vi "OriginalDigitizerLive - Copy (2).vi"() -> ()   [LabVIEW 2020]
doc: "Example Description:\nThis example demonstrates how to enable Time Interleaved Sampling with the NI 5772 adapter module to achieve a sampling rate of 1.6GS/s. This example continuously acquires records of analog input data from the NI 5772 adapter module. It allows you to select an AI channel, trigger type, and record size. This VI must be compiled before it is run. \n\nRunning the VI:\nThis VI must be run from the NI 5772 - Getting Started (Host).vi. Refer to the host VI documentation for steps regarding running and configuring the FPGA VI. \n\nExecution Steps:\nRefer to the Block Diagram of this VI for execution comments."
uses:
  Controls/AI Trigger Type.ctl
  Controls/Aquire State.ctl
  Controls/NeighbouringAvgStates.ctl
  <vilib>/Platform/TimedLoop/XDataNode/timing_clust.ctl
  <vilib>/Platform/TimedLoop/XDataNode/nitl_modes.ctl
  <vilib>/Platform/TimedLoop/XDataNode/wakeup.ctl
  <vilib>/rvi/Emulation/niFpgaGetClockAttributes.vi
  <vilib>/rvi/Emulation/niFpgaSctlEmulationGetInTimedLoop.vi
  <vilib>/rvi/Emulation/niFpgaEmulationReportErrorSimple.vi
  <vilib>/rvi/Emulation/niFpgaProcessEmulError.vi
  <vilib>/rvi/eio/common/nirviEmuTemplateMethod_errors.vi
  <vilib>/rvi/Emulation/niFpgaCriticalErrorInLSC.vi
  <vilib>/rvi/interface/RandomDataEmulation/niFpgaRandomDataHandleErrors.vi
  <vilib>/rvi/Emulation/niFpgaEmulationIsFPGAContextNoSignature.vi
  <vilib>/rvi/errors/niFpgaSetErrorForExecOnDevCompSimple.vi
  <vilib>/rvi/eio/common/nirviEmuReportErrorAndStop.vi
  <vilib>/rvi/DataTransferAndStorage/Container/Common/niFpgaContainerGetUniqueNameForEmu.vi
  <vilib>/rvi/FIFO/Fifo_Resource/nirvififoEmulationSetSize.vi
  <vilib>/rvi/FIFO/Fifo_Resource/nirviFifoEmulationQueueMgr.vi
  <instcachedir>/0/nirviFifoEmulationQueueMgr_E5CAEC123FF24DC58D834DCA3CDAA9B5.lvgen/nirviFifoEmulationQueueMgr_E5CAEC123FF24DC58D834DCA3CDAA9B5_000.vi
  <vilib>/Utility/error.llb/Clear Errors.vi
  <vilib>/rvi/FIFO/Fifo_Resource/nirvififoEmulationCreateLock.vi
  <vilib>/rvi/FIFO/Fifo_Resource/nirvififoEmulationObtainLock.vi
  <vilib>/rvi/FIFO/Fifo_Resource/nirvififoEmulationReleaseLock.vi
  <vilib>/rvi/occurrence/nirviWaitOnOccurrenceBase.vi
  <vilib>/rvi/errors/nirviReportUnexpectedCaseInternalError.vi
  <vilib>/rvi/errors/nirviReportUnexpectedCaseInternalError (U32).vi
  <vilib>/rvi/FIFO/Fifo_Resource/nirvififoEmulationDetermineInputValidOut.vi
  <vilib>/eio/EIONode/EIONode.xnode
  <vilib>/Platform/TimedLoop/XDataNode/XDataNode.xnode
  <vilib>/rvi/DataTransferAndStorage/Container/XNode/niFpgaContainer.xnode
  <vilib>/rvi/interface/RandomDataEmulation/nirviRandomDataFpgaReadWriteTemplate.vi
  <vilib>/rvi/FIFO/Fifo_Resource/nirvififoEmulationRead.vi
  <vilib>/rvi/FIFO/Fifo_Resource/nirvififoEmulationWrite.vi
  <vilib>/Platform/TimedLoop/XDataNode/XDNodeRunTimeDep.lvlib
  <instrlib>/_niInstr/Basic Elements/v1/FPGA/niInstr Basic Elements v1 FPGA.lvlib
  Controls/DigitizerState.ctl
  <vilib>/rvi/Memory/Memory_Emulation/nirvimemoryEmulation.vi
  <vilib>/rvi/Memory/Memory_Emulation/nirvimemoryFastEmulation.vi
panel:
  in  "Recording":bool
  in  "WaitForWave\nCompletion [cycles]":u16
  out "F to H FIFO Overflow?":bool caption="FIFO Overflow?"
  out "AvgCount":u16=1
  in  "AvgCount_powerOf2":i16=1
  in  "DS":u8
  in  "Trigger":bool=TRUE
  out "Acquire State":T1
  in  "Delay Cycles":u16=512 caption="Samples Per Trigger" min=1 step=1
  out "TS FIFO In Overflow?":bool caption="FIFO Overflow?"
  in  "Samples Per Trigger":u16=512 min=1 step=1
  in  "Arm Trigger":bool
  in  "User Command Commit":bool
  in  "User Command":u8
  out "User Command Idle":bool
  out "User Command Status":u8
  in  "User Data 0":u16
  in  "User Data 1":u8
  out "PLL Locked":bool
  out "User Error":bool
  out "Configured?":bool
  out "DMA FIFO Overflow?":bool caption="FIFO Overflow?"
  in  "Trigger Level":i16
  in  "Trigger Type":T2
  # "Resource Configuration"
  # "Refer to the Block Diagram of this VI for execution comments."
  # "For other instructions, select Help>>Show Context Help and move the cursor over the VI icon to display help for this VI."
  # "Analog Input"
  # "Clock Configuration"
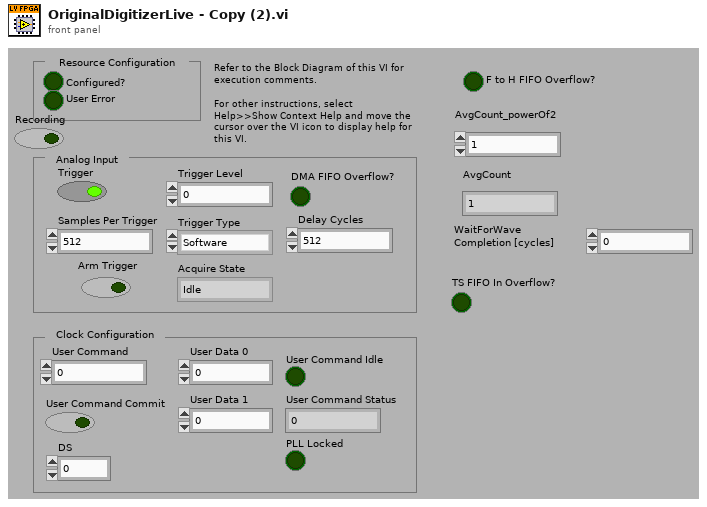
[diagram p1: front panel]
types:
  T1 = typedef "Aquire State.ctl" = enum8{"Idle", "Wait for Trigger", "AlignWave", "Hold Aquire", "Acquire", "WaitForWaveCompletion", "CheckAvg"}
  T2 = typedef "AI Trigger Type.ctl" = enum8{"Software", "Data Edge"}
  T3 = typedef "NeighbouringAvgStates.ctl" = enum16{"Read_noDS", "Write1_noDS", "Write2_noDS"}
  T4 = typedef "DigitizerState.ctl" = enum16{"Init", "Build/Clear Accumulator", "GetData", "SetData", "AverageCountCheck", "SendtoHost"}
  T5 = typedef "XDNodeRunTimeDep.lvlib/timing_clust.ctl" = cluster{"Expected End [f-1]":u64, "Actual End [f-1]":u64, "Finished Late? [f-1]":bool, "Expected End [i-1]":u64, "Actual End [i-1]":u64, "Finished Late? [i-1]":bool, "Expected Start [i]":u64, "Actual Start [i]":u64, "Expected Start [f]":u64, "Actual Start [f]":u64, "Source Name":string, "Structure Name":string, "Period":i64, "Deadline":i64, "Offset":i64, "Start":i64, "Priority":i32, "Timeout":i32, "Mode":T6, "Wakeup Reason":T7, "Error":errorcluster, "Source Type":string, "Secondary Source Type":string, "Global End Time":u64, "Global Start Time":u64, "Frame Duration":u64, "Iteration Duration":u64, "Assigned CPU":i32, "I/O Scan Engine Mode":u32}
  T6 = typedef "XDNodeRunTimeDep.lvlib/nitl_modes.ctl" = enum32{"No Change", "Process missed periods, maintain original phase", "Discard missed periods, maintain original phase", "Process missed periods, ignore original phase", "Discard missed periods, ignore original phase"}
  T7 = typedef "XDNodeRunTimeDep.lvlib/wakeup.ctl" = enum32{"Normal", "Aborted", "Asynchronous wakeup", "Timing source error", "Timed loop error", "Timeout"}
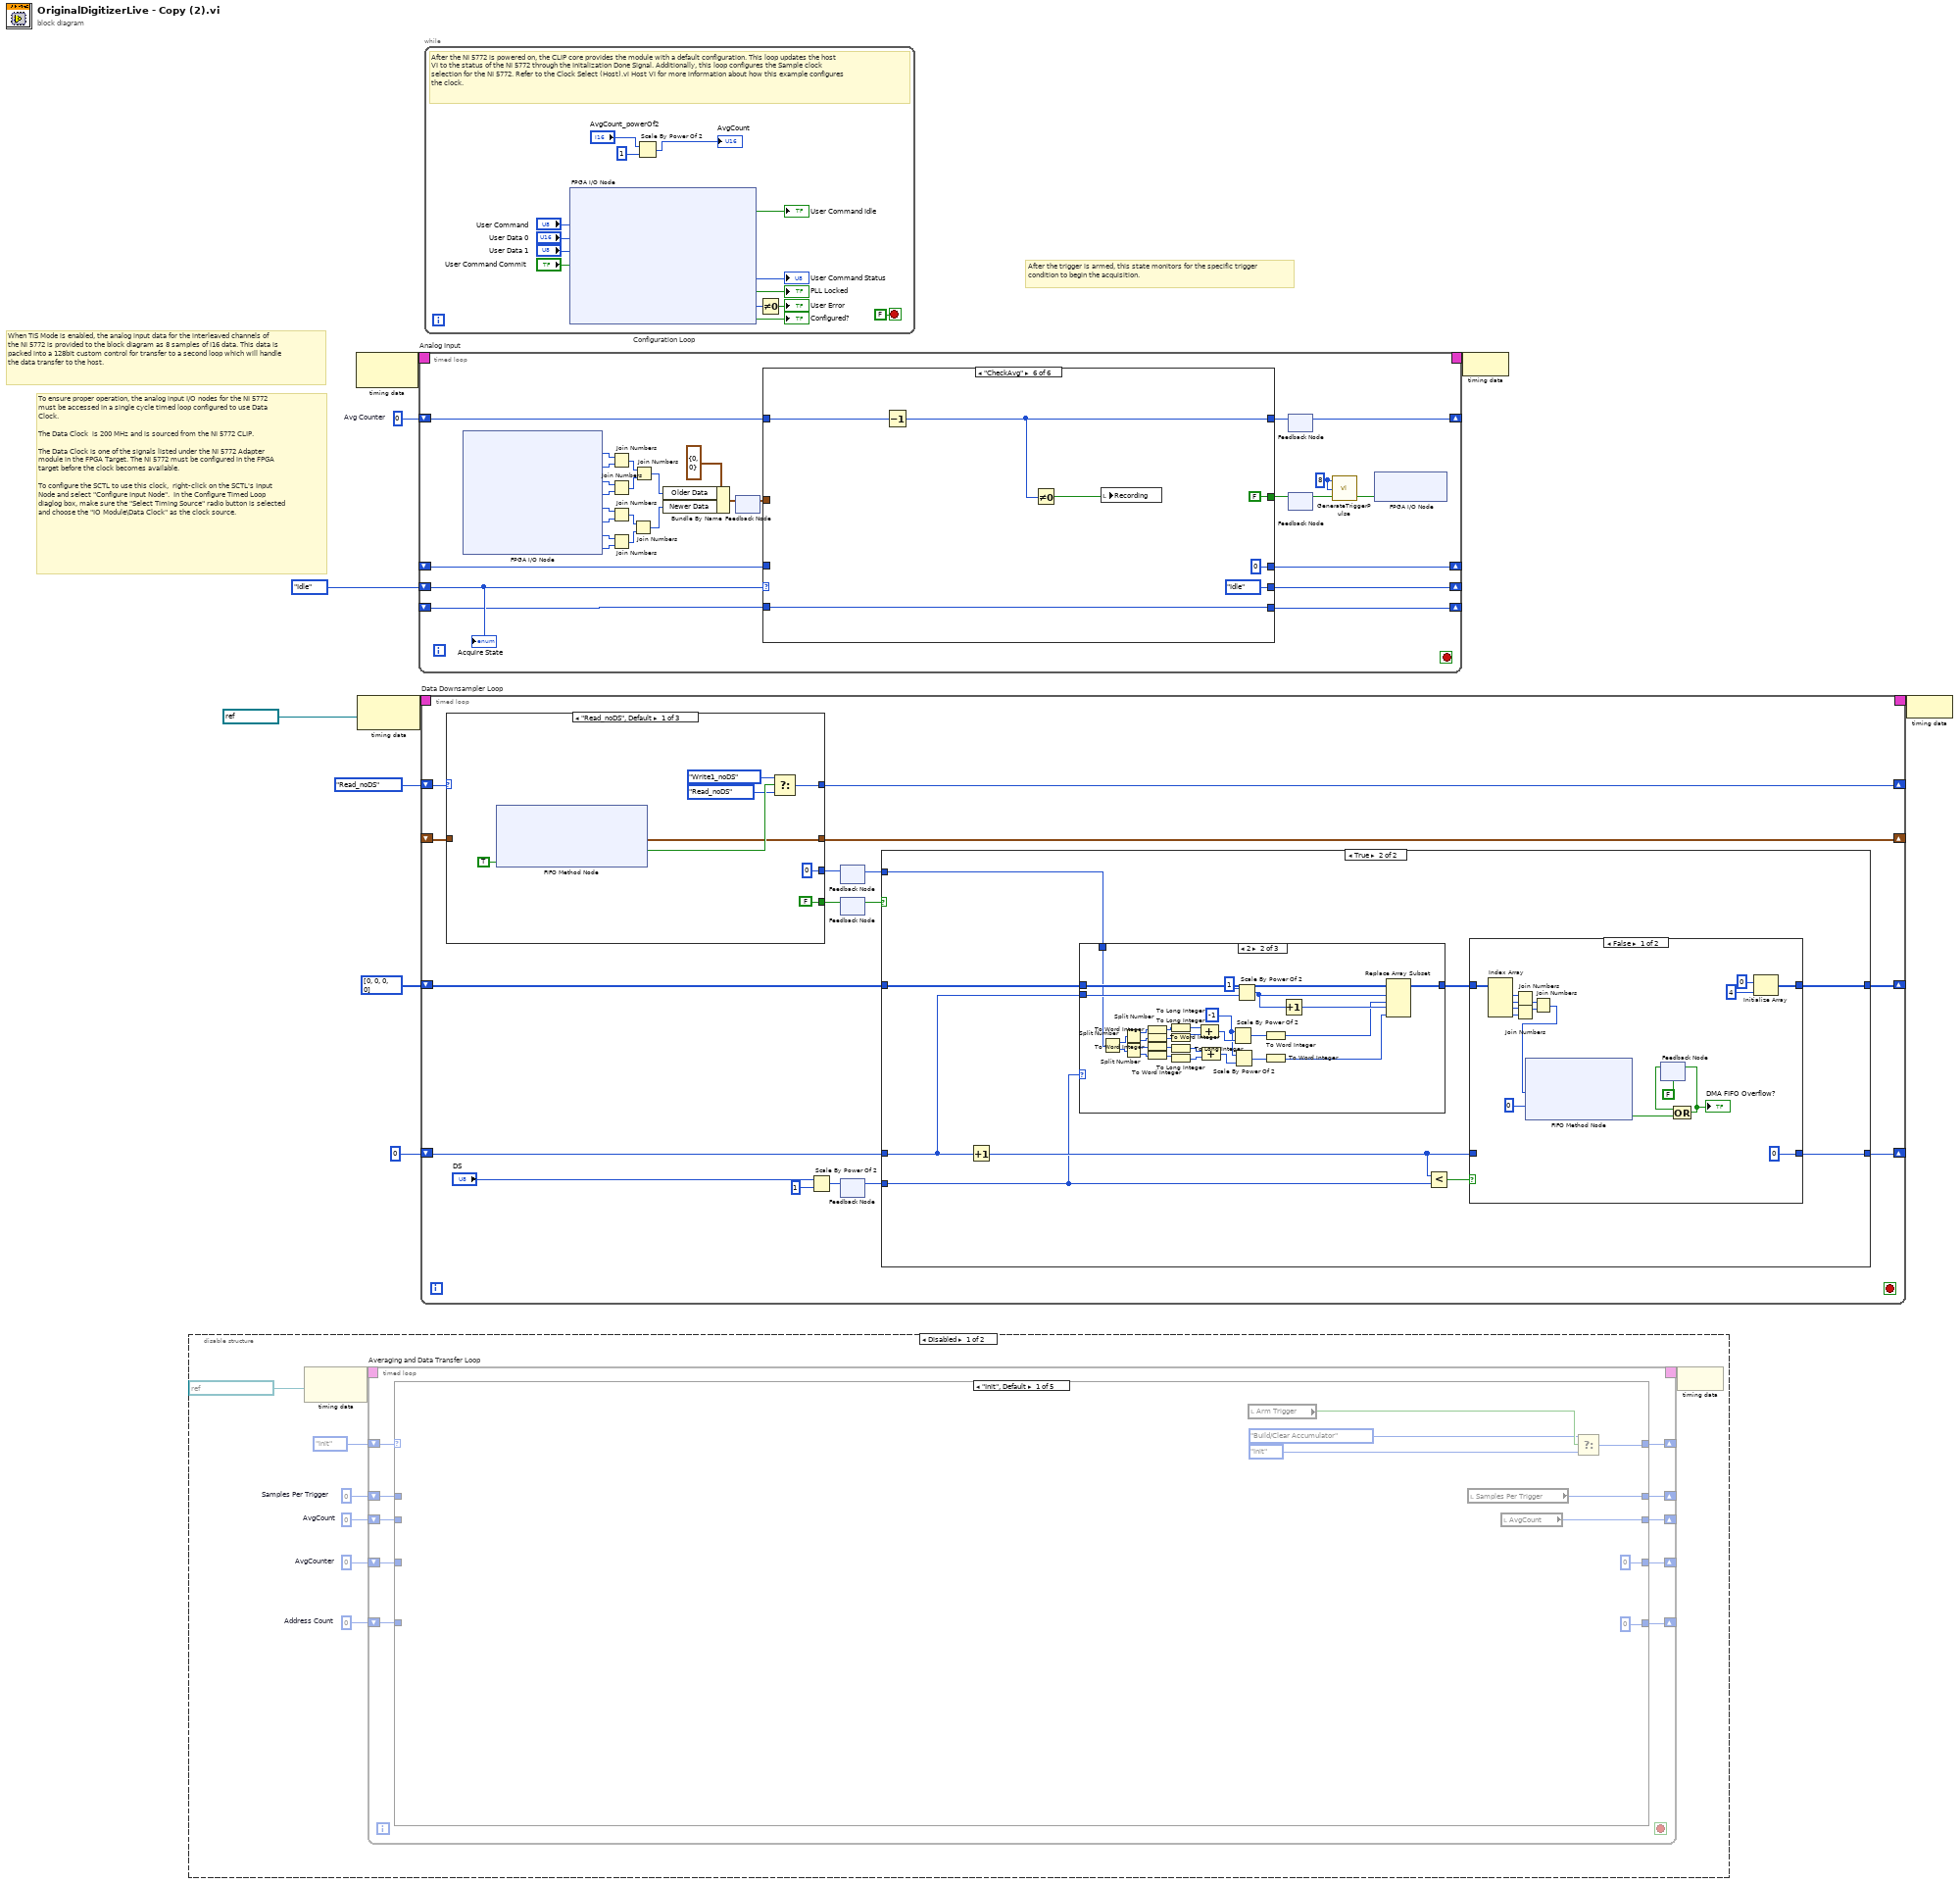
[diagram p0: block diagram]
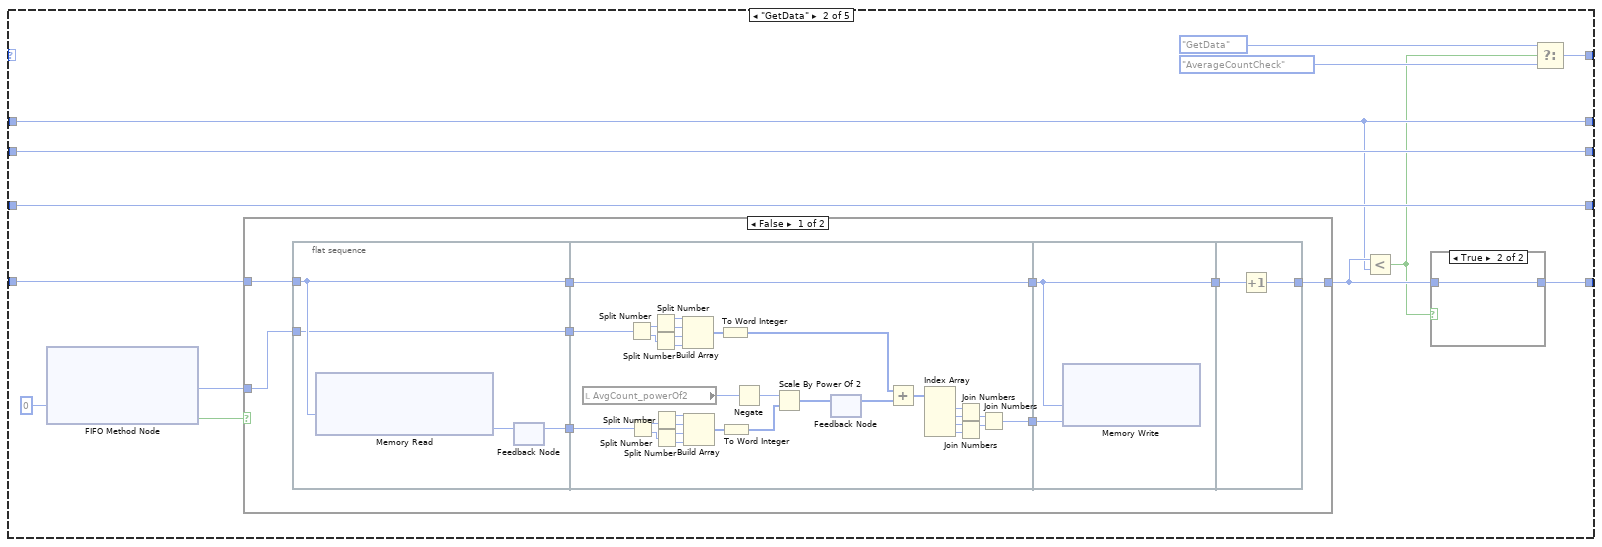
[diagram p2: hidden frame]
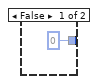
[diagram p3: hidden frame]
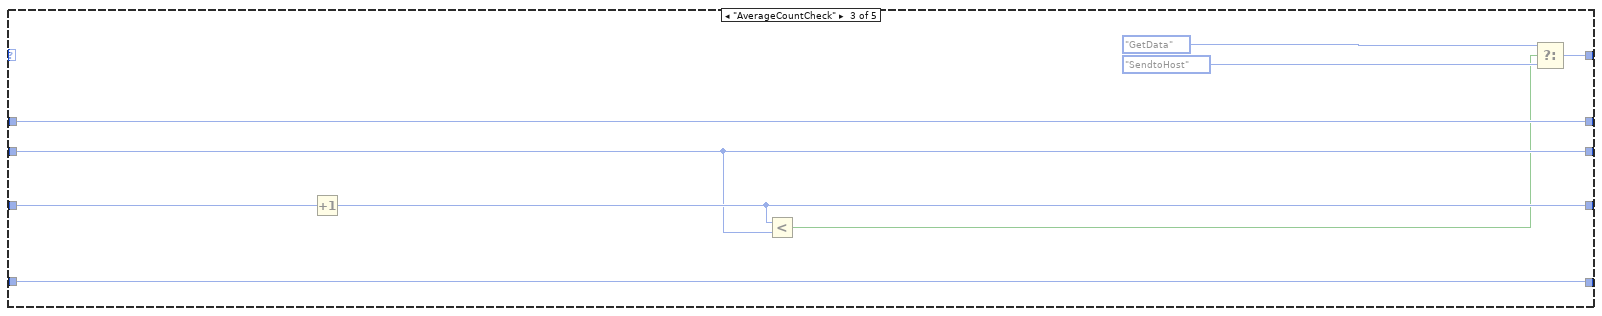
[diagram p5: hidden frame]
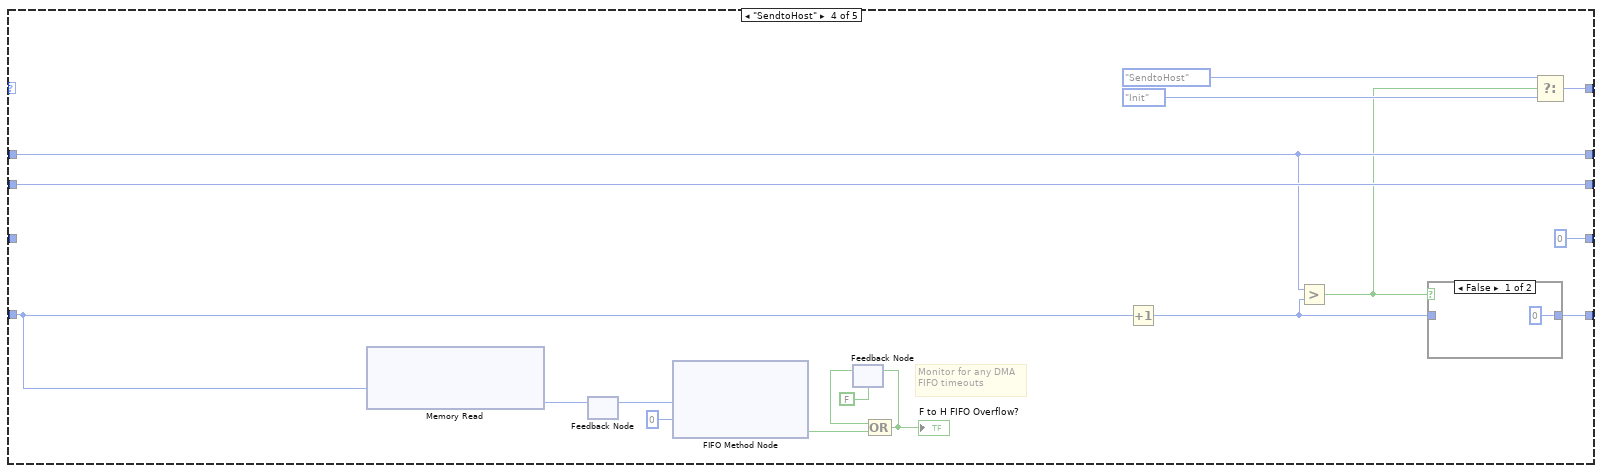
[diagram p6: hidden frame]
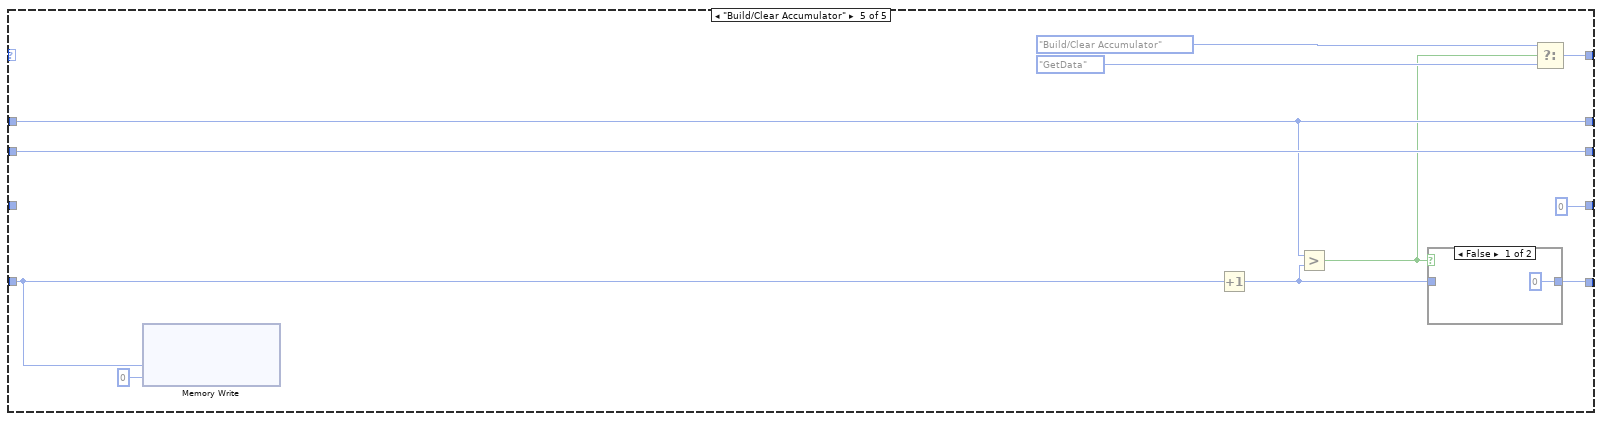
[diagram p8: hidden frame]
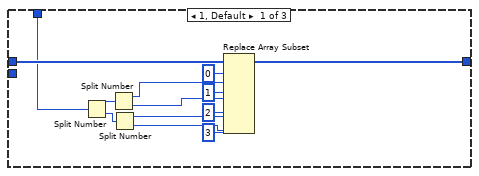
[diagram p13: hidden frame]
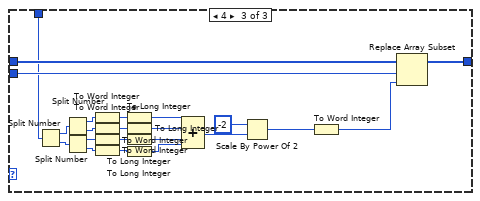
[diagram p14: hidden frame]
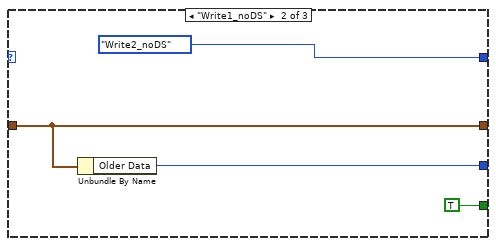
[diagram p15: hidden frame]
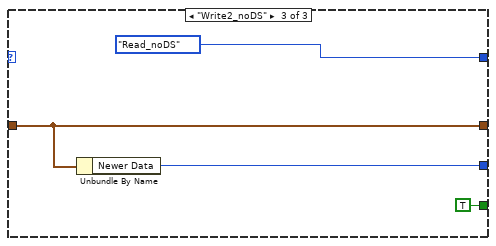
[diagram p16: hidden frame]
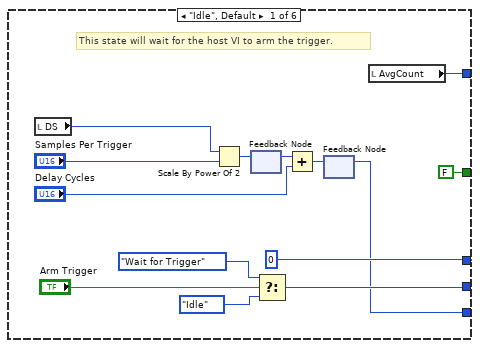
[diagram p17: hidden frame]
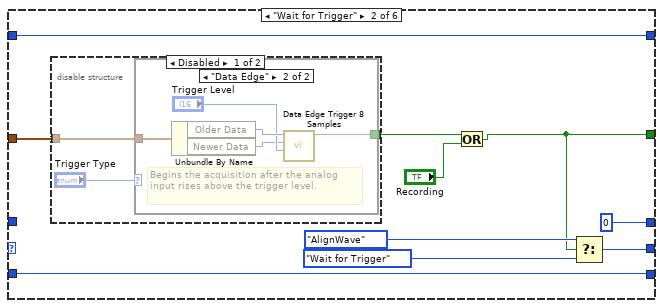
[diagram p18: hidden frame]
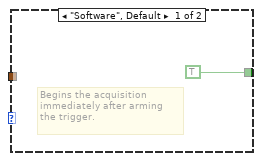
[diagram p19: hidden frame]
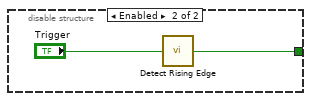
[diagram p20: hidden frame]
diagram:
  w1 = u16 0  # Avg Counter
  # "After the trigger is armed, this state monitors for the specific trigger condition to begin the acquisition."
  # "When TIS Mode is enabled, the analog input data for the interleaved channels of the NI 5772 is provided to the block diagram as 8 samples of I16 data. This data is packed into a 128bit custom control for transfer to a second loop which will handle the data transfer to the host."
  # "To ensure proper operation, the analog input I/O nodes for the NI 5772 must be accessed in a single cycle timed loop configured to use Data Clock. \n\nThe Data Clock  is 200 MHz and is sourced from the NI 5772 CLIP.\n\nThe Data Clock is one of the signals listed under the NI 5772 Adapter module in the FPGA Target. The NI 5772 must be configured in the FPGA target before the clock becomes available. \n\nTo configure the SCTL to use this clock,  right-click on the SCTL's Input Node and select \"Configure Input Node\".  In the Configure Timed Loop diaglog box, make sure the \"Select Timing Source\" radio button is selected and choose the \"IO Module\\Data Clock\" as the clock source."
  n1 = disable-structure shown="Disabled" {
    frame Disabled {
      w16 = u16 0  # AvgCounter
      w15 = u32 0  # Address Count
      w14 = u16 0  # AvgCount
      w13 = u16 0  # Samples Per Trigger
      n2 = node-c288(refnum<k21> "200 MHz Clock" ("Source Name")) -> (w18:T5)
      n3 = timed-loop "Averaging and Data Transfer Loop" {
        timing: w18 -> [_]
        timing-out: [_] -> w17
        shift-right: [w27] -> _
        shift-left: DigitizerState."Init" -> [w28]
        shift-right: [w26] -> _
        shift-left: w13 -> [w24]
        shift-right: [w25] -> _
        shift-left: w14 -> [w23]
        shift-right: [w21] -> _
        shift-left: w15 -> [w22]
        shift-right: [w19] -> _
        shift-left: w16 -> [w20]
        stop <- _ stop-if-true
        n4 = case shown="\"Init\", Default" w28 {
          tunnel: [w32 w47 w107 w123 w136] -> w27
          tunnel: [w30 w39 w105 w121 w134] -> w26
          tunnel: [w33 w46 w102 w126 w139] -> w25
          tunnel: w24 -> [_ w39 w105 w121 w134]
          tunnel: w23 -> [_ w46 w102 w126 w139]
          tunnel: w22 -> [_ w42 w106 w111 w130]
          tunnel: [u32 0 w41 w106 w122 w135] -> w21
          tunnel: [u16 0 w44 w103 u16 0 ("AvgCounter") u16 0 ("AvgCounter")] -> w19
          tunnel: w20 -> [_ w44 w104 _ _]
          frame "Init", Default {
            n5 = local read "Arm Trigger"() -> (w36:bool)
            n6 = local read "Samples Per Trigger"() -> (w30:u16)
            n7 = local read "AvgCount"() -> (w33:u16)
            n8 = Select(t=DigitizerState."Build/Clear Accumulator", s=w36, f=DigitizerState."Init") -> (s? t:f=w32:T4)
          }
          frame "GetData" {
            n9 = xnode ("FIFO Method Node")("Timeout"=0) -> ("Element"=w43:u64, "Timed Out?"=w38:bool)  [unwired: 1 in, 1 out]
            n10 = case shown="False" w38 {
              tunnel: w43 -> [w57 _]
              tunnel: w42 -> [w59 w100]
              tunnel: [w56 w100] -> w40
              frame False {
                n11 = flat-sequence {
                  tunnel: [w63] -> w60
                  tunnel: w59 -> [w62]
                  tunnel: w57 -> [w61]
                  tunnel: [w62] -> w55
                  tunnel: [w61] -> w53
                  tunnel: w60 -> [w66]
                  tunnel: [w85] -> w58
                  tunnel: w55 -> [w84]
                  tunnel: [w84] -> w54
                  tunnel: w53 -> [w75]
                  tunnel: w58 -> [w97]
                  tunnel: w54 -> [w96]
                  tunnel: [w96] -> w52
                  tunnel: [w98] -> w56
                  tunnel: w52 -> [w99]
                  frame #0 {
                    n12 = xnode ("Memory Read")("Address"=w62) -> ("Data"=w64:u64)  [unwired: 1 in, 1 out]
                    n13 = feedback #1() -> (w63:u64)  [unwired: 1 in]
                    n14 = feedback-in #1(w64) -> ()
                  }
                  frame #1 {
                    n15 = local read "AvgCount_powerOf2"() -> (w94:i16)
                    n16 = Split Number(x=w75) -> (hi(x)=w82:u32, lo(x)=w81:u32)
                    n17 = Split Number(x=w66) -> (hi(x)=w67:u32, lo(x)=w68:u32)
                    n18 = Split Number(x=w82) -> (hi(x)=w80:u16, lo(x)=w79:u16)
                    n19 = Split Number(x=w81) -> (hi(x)=w78:u16, lo(x)=w77:u16)
                    n20 = Split Number(x=w67) -> (hi(x)=w69:u16, lo(x)=w70:u16)
                    n21 = Split Number(x=w68) -> (hi(x)=w71:u16, lo(x)=w72:u16)
                    n22 = Build Array(w80, w79, w78, w77) -> (w76:u16[])
                    n23 = Build Array(w69, w70, w71, w72) -> (w73:u16[])
                    n24 = To Word Integer(number=w76) -> (16bit integer=w74:i16[])
                    n25 = To Word Integer(number=w73) -> (16bit integer=w65:i16[])
                    n26 = Negate(x=w94) -> (-x=w95:i16)
                    n27 = Scale By Power Of 2(n=w95, x=w65) -> (x*2^n=w93:i16[])
                    n28 = feedback-in #2(w93) -> ()
                    n29 = feedback #2() -> (w83:i16[])  [unwired: 1 in]
                    n30 = Add(x=w74, y=w83) -> (x+y=w86:i16[])
                    n31 = Index Array(array=w86) -> (element #1=w89:i16, element #2=w90:i16, element #3=w91:i16, element #4=w92:i16)  [unwired: 4 in]
                    n32 = Join Numbers(hi=w89, lo=w90) -> ((hi.lo)=w87:u32)
                    n33 = Join Numbers(hi=w91, lo=w92) -> ((hi.lo)=w88:u32)
                    n34 = Join Numbers(hi=w87, lo=w88) -> ((hi.lo)=w85:u64)
                  }
                  frame #2 {
                    n35 = xnode ("Memory Write")("Address"=w96, "Data"=w97) -> ()  [unwired: 1 in, 1 out]
                  }
                  frame #3 {
                    n36 = Increment(x=w99) -> (x+1=w98:u32)
                  }
                }
              }
              frame True {
              }
            }
            n37 = Less?(x=w40, y=w39) -> (x < y?=w37:bool)
            n38 = case shown="True" w37 {
              tunnel: w40 -> [_ w51]
              tunnel: [u32 0 w51] -> w41
              frame False {
              }
              frame True {
              }
            }
            n39 = Select(t=DigitizerState."GetData", s=w37, f=DigitizerState."AverageCountCheck") -> (s? t:f=w47:T4)
          }
          frame "AverageCountCheck" {
            n40 = Increment(x=w104) -> (x+1=w103:u16)
            n41 = Less?(x=w103, y=w102) -> (x < y?=w101:bool)
            n42 = Select(t=DigitizerState."GetData", s=w101, f=DigitizerState."SendtoHost") -> (s? t:f=w107:T4)
          }
          frame "SendtoHost" {
            # "Monitor for any DMA FIFO timeouts"
            n43 = xnode ("Memory Read")("Address"=w111) -> ("Data"=w112:u64)  [unwired: 1 in, 1 out]
            n44 = feedback #3() -> (w110:u64)  [unwired: 1 in]
            n45 = feedback-in #3(w112) -> ()
            n46 = xnode ("FIFO Method Node")("Element"=w110, "Timeout"=0) -> ("Timed Out?"=w117:bool)  [unwired: 1 in, 1 out]
            n47 = feedback #4(FALSE) -> (w116:bool)
            n48 = Compound Arithmetic op=OR(w116, w117) -> (w118:bool)
            "F to H FIFO Overflow?" <- w118
            n49 = feedback-in #4(w118) -> ()
            n50 = Increment(x=w111) -> (x+1=w120:u32)
            n51 = Greater?(x=w121, y=w120) -> (0:w119:bool)
            n52 = case shown="False" w119 {
              tunnel: w120 -> [_ w128]
              tunnel: [u32 0 w128] -> w122
              frame False {
              }
              frame True {
              }
            }
            n53 = Select(t=DigitizerState."SendtoHost", s=w119, f=DigitizerState."Init") -> (s? t:f=w123:T4)
          }
          frame "Build/Clear Accumulator" {
            n54 = xnode ("Memory Write")("Address"=w130, "Data"=u64 0) -> ()  [unwired: 1 in, 1 out]
            n55 = Increment(x=w130) -> (x+1=w133:u32)
            n56 = Greater?(x=w134, y=w133) -> (0:w132:bool)
            n57 = case shown="False" w132 {
              tunnel: w133 -> [_ w141]
              tunnel: [u32 0 w141] -> w135
              frame False {
              }
              frame True {
              }
            }
            n58 = Select(t=DigitizerState."Build/Clear Accumulator", s=w132, f=DigitizerState."GetData") -> (s? t:f=w136:T4)
          }
        }
      }
      n59 = node-c288(w17) -> ()
    }
    frame Enabled {
    }
  }
  n60 = node-c288() -> (w10:T5)  [unwired: 1 in]
  n61 = node-c288(refnum<k21> "160MHz" ("Source Name")) -> (w6:T5)
  n62 = timed-loop "Analog Input" {
    timing: w10 -> [_]
    timing-out: [_] -> w9
    shift-right: [w176] -> _
    shift-left: Aquire_State."Idle" ("Acquire State") -> [w166]
    shift-right: [w177] -> _
    shift-left: _ -> [w167]
    shift-right: [w175] -> _
    shift-left: _ -> [w165]
    shift-right: [w148] -> _
    shift-left: w1 -> [w151]
    stop <- _ stop-if-true
    w153 = u16 8 ("Pulse Width On [cycles]")
    n63 = xnode "FPGA I/O Node"() -> ("IO Module\\AI 1 Data N-3"=w158:i16, "IO Module\\AI 0 Data N-3"=w157:i16, "IO Module\\AI 1 Data N-2"=w156:i16, "IO Module\\AI 0 Data N-2"=w155:i16, "IO Module\\AI 1 Data N-1"=w159:i16, "IO Module\\AI 0 Data N-1"=w160:i16, "IO Module\\AI 1 Data N"=w161:i16, "IO Module\\AI 0 Data N"=w162:i16)  [unwired: 8 in, 8 out]
    n64 = Join Numbers(hi=w158, lo=w157) -> ((hi.lo)=w170:u32)
    n65 = Join Numbers(hi=w156, lo=w155) -> ((hi.lo)=w172:u32)
    n66 = Join Numbers(hi=w159, lo=w160) -> ((hi.lo)=w171:u32)
    n67 = Join Numbers(hi=w161, lo=w162) -> ((hi.lo)=w173:u32)
    n68 = Join Numbers(hi=w171, lo=w173) -> ((hi.lo)=w163:u64)
    n69 = Join Numbers(hi=w170, lo=w172) -> ((hi.lo)=w164:u64)
    n70 = Bundle By Name(cluster=cluster{"Older Data":u64, "Newer Data":u64} {"Older Data"=0, "Newer Data"=0} ("Element"), "Older Data"=w164, "Newer Data"=w163) -> (w168:cluster{"Older Data":u64, "Newer Data":u64})
    n71 = feedback #5() -> (w174:cluster{"Older Data":u64, "Newer Data":u64})  [unwired: 1 in]
    n72 = feedback-in #5(w168) -> ()
    n73 = case shown="\"CheckAvg\"" w166 {
      tunnel: [u16 0 u16 0 w217 w226 w249 u16 0 ("f")] -> w177
      tunnel: w167 -> [_ _ w217 w240 w247 _]
      tunnel: [w188 w197 w218 w239 w244 Aquire_State."Idle" ("Acquire State")] -> w176
      tunnel: [w185 w201 w216 w236 w250 w256] -> w175
      tunnel: w165 -> [_ w201 w216 w236 w250 w256]
      tunnel: w174 -> [_ w200 _ w235 _ _]
      tunnel: [FALSE ("edge detected") w193 FALSE ("edge detected") FALSE ("edge detected") FALSE ("edge detected") FALSE ("edge detected")] -> w152
      tunnel: w151 -> [_ w194 w214 w222 w242 w257]
      tunnel: [w179 w194 w214 w222 w242 w254] -> w150
      frame "Idle", Default {
        # "This state will wait for the host VI to arm the trigger."
        n74 = local read "DS"() -> (w181:u8)
        n75 = Scale By Power Of 2(n=w181, x="Samples Per Trigger") -> (x*2^n=w183:u16)
        n76 = feedback-in #6(w183) -> ()
        n77 = feedback #6() -> (w180:u16)  [unwired: 1 in]
        n78 = Select(t=Aquire_State."Wait for Trigger" ("Acquire State"), s="Arm Trigger", f=Aquire_State."Idle" ("Acquire State")) -> (s? t:f=w188:T1)
        n79 = Add(x=w180, y="Delay Cycles") -> (x+y=w186:u16)
        n80 = feedback-in #7(w186) -> ()
        n81 = feedback #7() -> (w185:u16)  [unwired: 1 in]
        n82 = local read "AvgCount"() -> (w179:u16)
      }
      frame "Wait for Trigger" {
        n83 = disable-structure shown="Disabled" {
          disable-tunnel: w200 -> [w203 _]
          disable-tunnel: [w202 w211] -> w195
          frame Disabled {
            n84 = case shown="\"Data Edge\"" "Trigger Type" {
              tunnel: w203 -> [_ w210]
              tunnel: [TRUE ("Trigger") w209] -> w202
              frame "Software", Default {
                # "Begins the acquisition immediately after arming the trigger."
              }
              frame "Data Edge" {
                # "Begins the acquisition after the analog input rises above the trigger level."
                n85 = Unbundle By Name(w210) -> ("Older Data"=w208:u64, "Newer Data"=w206:u64)
                n86 = call "Data Edge Trigger 8 Samples.vi"("Trigger Level"="Trigger Level", "Newer Data In"=w206, "Older Data In"=w208) -> ("Trigger"=w209:bool)  [unwired: 8 in]
              }
            }
          }
          frame Enabled {
            n87 = call <instrlib>:"Detect Rising Edge.vi"("signal"="Trigger") -> ("edge detected"=w211:bool)  [unwired: 14 in]
          }
        }
        n88 = Or(x=w195, y="Recording") -> (x .or. y?=w193:bool)
        n89 = Select(t=Aquire_State."AlignWave" ("Acquire State"), s=w193, f=Aquire_State."Wait for Trigger") -> (s? t:f=w197:T1)
      }
      frame "AlignWave" {
        n90 = xnode "FPGA I/O Node"() -> ("PXI_Trig0"=w215:bool)  [unwired: 1 in, 1 out]
        n91 = Select(t=Aquire_State."Acquire" ("Acquire State"), s=w215, f=Aquire_State."AlignWave") -> (s? t:f=w218:T1)
      }
      frame "Acquire" {
        # "Monitor for any  FIFO timeouts"
        # "While in this state, data is pushed into a DMA FIFO until the desired number of samples per record have been acquired."
        n92 = local read "Delay Cycles"() -> (w234:u16)
        n93 = Increment(x=w240) -> (x+1=w225:u16)
        n94 = Less?(x=w234, y=w225) -> (x < y?=w230:bool)
        n95 = feedback-in #8(w230) -> ()
        n96 = feedback #8() -> (w227:bool)  [unwired: 1 in]
        n97 = Less?(x=w225, y=w236) -> (x < y?=w224:bool)
        n98 = xnode ("FIFO Method Node")("Element"=w235, "Input Valid"=w227) -> ("Ready for Input"=w229:bool)  [unwired: 1 in, 1 out]
        n99 = Not(x=w229) -> (.not. x?=w228:bool)
        n100 = feedback #9(FALSE) -> (w231:bool)
        n101 = Or(x=w231, y=w228) -> (x .or. y?=w232:bool)
        "TS FIFO In Overflow?" <- w232
        n102 = feedback-in #9(w232) -> ()
        n103 = Select(t=Aquire_State."Acquire" ("Acquire State"), s=w224, f=Aquire_State."WaitForWaveCompletion" ("Acquire State")) -> (s? t:f=w239:T1)
        n104 = Select(t=w225, s=w224, f=u16 0) -> (s? t:f=w226:u16)
      }
      frame "WaitForWaveCompletion" {
        n105 = Greater?(x="WaitForWave\nCompletion [cycles]", y=w247) -> (0:w243:bool)
        n106 = Increment(x=w247) -> (x+1=w249:u16)
        n107 = Select(t=Aquire_State."WaitForWaveCompletion" ("Acquire State"), s=w243, f=Aquire_State."CheckAvg" ("Acquire State")) -> (s? t:f=w244:T1)
      }
      frame "CheckAvg" {
        n108 = Decrement(x=w257) -> (x-1=w254:u16)
        n109 = Not Equal To 0?(x=w254) -> (x != 0?=w252:bool)
        n110 = local write "Recording"(w252) -> ()
      }
    }
    n111 = feedback-in #10(w150) -> ()
    n112 = feedback #10() -> (w148:u16)  [unwired: 1 in]
    n113 = feedback-in #11(w152) -> ()
    n114 = feedback #11() -> (w149:bool)  [unwired: 1 in]
    n115 = call "GenerateTriggerPulse.vi"("Trigger"=w149, "Pulse Width Off [cycles]"=w153, "Pulse Width On [cycles]"=w153) -> ("Out"=w154:bool)  [unwired: 2 out]
    n116 = xnode "FPGA I/O Node"("PXI_Trig1"=w154) -> ()  [unwired: 1 in, 1 out]
    "Acquire State" <- w166
  }
  n117 = timed-loop "Data Downsampler Loop" {
    shift-right: [w274] -> _
    shift-left: NeighbouringAvgStates."Read_noDS" -> [w275]
    timing: w6 -> [_]
    timing-out: [_] -> w5
    shift-right: [w273] -> _
    shift-left: _ -> [w272]
    shift-right: [w262] -> _
    shift-left: u16 0 -> [w263]
    shift-right: [w260] -> _
    shift-left: i16[] [0, 0, 0, 0] -> [w261]
    stop <- _ stop-if-true
    n118 = case shown="\"Read_noDS\", Default" w275 {
      tunnel: [w375 NeighbouringAvgStates."Write2_noDS" ("f") NeighbouringAvgStates."Read_noDS" ("f")] -> w274
      tunnel: [w371 w379 w383] -> w273
      tunnel: w272 -> [_ w379 w383]
      tunnel: [u64 0 ("Newer Data") w378 w382] -> w270
      tunnel: [FALSE ("Input Valid") TRUE ("Input Valid") TRUE ("Input Valid")] -> w271
      frame "Read_noDS", Default {
        n119 = xnode ("FIFO Method Node")("Ready for Output"=TRUE) -> ("Element"=w371:cluster{"Older Data":u64, "Newer Data":u64}, "Output Valid"=w374:bool)  [unwired: 1 in, 1 out]
        n120 = Select(t=NeighbouringAvgStates."Write1_noDS", s=w374, f=NeighbouringAvgStates."Read_noDS") -> (s? t:f=w375:T3)
      }
      frame "Write1_noDS" {
        n121 = Unbundle By Name(w379) -> ("Older Data"=w378:u64)
      }
      frame "Write2_noDS" {
        n122 = Unbundle By Name(w383) -> ("Newer Data"=w382:u64)
      }
    }
    n123 = Scale By Power Of 2(n="DS", x=u8 1) -> (x*2^n=w268:u8)
    n124 = feedback-in #12(w270) -> ()
    n125 = feedback #12() -> (w265:u64)  [unwired: 1 in]
    n126 = feedback-in #13(w271) -> ()
    n127 = feedback #13() -> (w264:bool)  [unwired: 1 in]
    n128 = feedback-in #14(w268) -> ()
    n129 = feedback #14() -> (w266:u8)  [unwired: 1 in]
    n130 = case shown="True" w264 {
      tunnel: w265 -> [_ w283]
      tunnel: w266 -> [_ w282]
      tunnel: w263 -> [w277 w281]
      tunnel: [w277 w280] -> w262
      tunnel: w261 -> [w276 w279]
      tunnel: [w276 w278] -> w260
      frame False {
      }
      frame True {
        n131 = Increment(x=w281) -> (x+1=w286:u16)
        n132 = case shown="2" w282 {
          tunnel: w279 -> [w318 w340 w362]
          tunnel: [w317 w339 w361] -> w285
          tunnel: w281 -> [_ w336 w360]
          tunnel: w283 -> [w306 w334 w355]
          frame 1, Default {
            n133 = Split Number(x=w306) -> (hi(x)=w316:u32, lo(x)=w315:u32)
            n134 = Split Number(x=w316) -> (hi(x)=w314:u16, lo(x)=w313:u16)
            n135 = Split Number(x=w315) -> (hi(x)=w312:u16, lo(x)=w311:u16)
            n136 = Replace Array Subset(array=w318, new element #1=w314, index #1=0 ("index"), new element #2=w313, index #2=1 ("index"), new element #3=w312, index #3=2 ("index"), new element #4=w311, index #4=3 ("index")) -> (w317:i16[])
          }
          frame 2 {
            w319 = i16 -1 ("n")
            n137 = Split Number(x=w334) -> (hi(x)=w346:u32, lo(x)=w345:u32)
            n138 = Split Number(x=w346) -> (hi(x)=w344:u16, lo(x)=w343:u16)
            n139 = Split Number(x=w345) -> (hi(x)=w342:u16, lo(x)=w341:u16)
            n140 = To Word Integer(number=w344) -> (16bit integer=w333:i16)
            n141 = To Word Integer(number=w343) -> (16bit integer=w331:i16)
            n142 = To Word Integer(number=w342) -> (16bit integer=w330:i16)
            n143 = To Word Integer(number=w341) -> (16bit integer=w332:i16)
            n144 = To Long Integer(number=w333) -> (32bit integer=w329:i32)
            n145 = To Long Integer(number=w331) -> (32bit integer=w328:i32)
            n146 = To Long Integer(number=w330) -> (32bit integer=w327:i32)
            n147 = To Long Integer(number=w332) -> (32bit integer=w326:i32)
            n148 = Compound Arithmetic op=ADD(w329, w328) -> (w320:i32)
            n149 = Compound Arithmetic op=ADD(w327, w326) -> (w321:i32)
            n150 = Scale By Power Of 2(n=w319, x=w320) -> (x*2^n=w322:i32)
            n151 = Scale By Power Of 2(n=w319, x=w321) -> (x*2^n=w323:i32)
            n152 = Scale By Power Of 2(n=i16 1, x=w336) -> (x*2^n=w337:u16)
            n153 = To Word Integer(number=w322) -> (16bit integer=w324:i16)
            n154 = To Word Integer(number=w323) -> (16bit integer=w325:i16)
            n155 = Increment(x=w337) -> (x+1=w338:u16)
            n156 = Replace Array Subset(array=w340, new element #1=w324, index #1=w337, new element #2=w325, index #2=w338) -> (w339:i16[])
          }
          frame 4 {
            n157 = Split Number(x=w355) -> (hi(x)=w368:u32, lo(x)=w367:u32)
            n158 = Split Number(x=w368) -> (hi(x)=w366:u16, lo(x)=w365:u16)
            n159 = Split Number(x=w367) -> (hi(x)=w364:u16, lo(x)=w363:u16)
            n160 = To Word Integer(number=w366) -> (16bit integer=w359:i16)
            n161 = To Word Integer(number=w365) -> (16bit integer=w358:i16)
            n162 = To Word Integer(number=w364) -> (16bit integer=w357:i16)
            n163 = To Word Integer(number=w363) -> (16bit integer=w356:i16)
            n164 = To Long Integer(number=w359) -> (32bit integer=w351:i32)
            n165 = To Long Integer(number=w358) -> (32bit integer=w352:i32)
            n166 = To Long Integer(number=w357) -> (32bit integer=w353:i32)
            n167 = To Long Integer(number=w356) -> (32bit integer=w354:i32)
            n168 = Compound Arithmetic op=ADD(w351, w352, w353, w354) -> (w350:i32)
            n169 = Scale By Power Of 2(n=i16 -2, x=w350) -> (x*2^n=w348:i32)
            n170 = To Word Integer(number=w348) -> (16bit integer=w347:i16)
            n171 = Replace Array Subset(array=w362, new element=w347, index=w360) -> (w361:i16[])
          }
        }
        n172 = Less?(x=w286, y=w282) -> (x < y?=w284:bool)
        n173 = case shown="False" w284 {
          tunnel: w285 -> [w297 w305]
          tunnel: [w294 w305] -> w278
          tunnel: w286 -> [_ w304]
          tunnel: [u16 0 w304] -> w280
          frame False {
            n174 = Index Array(array=w297) -> (element #1=w301:i16, element #2=w300:i16, element #3=w299:i16, element #4=w298:i16)  [unwired: 4 in]
            n175 = Join Numbers(hi=w301, lo=w300) -> ((hi.lo)=w303:u32)
            n176 = Join Numbers(hi=w299, lo=w298) -> ((hi.lo)=w302:u32)
            n177 = Join Numbers(hi=w303, lo=w302) -> ((hi.lo)=w288:u64)
            n178 = xnode ("FIFO Method Node")("Element"=w288, "Timeout"=0) -> ("Timed Out?"=w289:bool)  [unwired: 1 in, 1 out]
            n179 = feedback #15(FALSE) -> (w290:bool)
            n180 = Compound Arithmetic op=OR(w290, w289) -> (w287:bool)
            "DMA FIFO Overflow?" <- w287
            n181 = feedback-in #15(w287) -> ()
            n182 = Initialize Array(i16 0 ("element"), 4 ("dimension size")) -> (w294:i16[])
          }
          frame True {
          }
        }
      }
    }
  }
  n183 = while "Configuration Loop" {
    stop <- FALSE stop-if-true
    # "After the NI 5772 is powered on, the CLIP core provides the module with a default configuration. This loop updates the host VI to the status of the NI 5772 through the Initalization Done Signal. Additionally, this loop configures the Sample clock selection for the NI 5772. Refer to the Clock Select (Host).vi Host VI for more information about how this example configures the clock."
    n184 = xnode "FPGA I/O Node"("IO Module\\User Command"="User Command", "IO Module\\User Data 0"="User Data 0", "IO Module\\User Data 1"="User Data 1", "IO Module\\User Command Commit"="User Command Commit") -> ("IO Module\\User Command Idle"=→"User Command Idle":bool, "IO Module\\User Command Status"=→"User Command Status":u8, "IO Module\\PLL Locked"=→"PLL Locked":bool, "IO Module\\User Error"=w395:u8, "IO Module\\Initialization Done"=→"Configured?":bool)  [unwired: 9 in, 9 out]
    n185 = Scale By Power Of 2(n="AvgCount_powerOf2", x=u16 1) -> (x*2^n=→"AvgCount":u16)
    n186 = Not Equal To 0?(x=w395) -> (x != 0?=→"User Error":bool)
  }
  n187 = node-c288(w9) -> ()
  n188 = node-c288(w5) -> ()
